vi "设置本机表.vi"(4 "本机表参数":cluster{"有功常数":i32, "无功常数":i32, "输出类型":i32}={"有功常数"=3600000, "无功常数"=3600000, "输出类型"=0}, 5 "串口号":refnum<visa-resource-name>) -> (1 "应答":string)   [LabVIEW 2014]
panel:
  in  "脉冲出口":u8
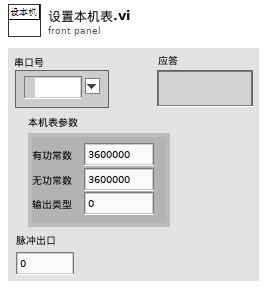
[diagram p1: front panel]
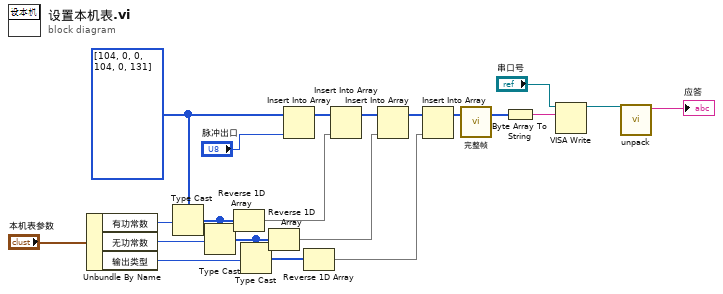
[diagram p0: block diagram]
diagram:
  w9 = u8[] [104, 0, 0, 104, 0, 131]
  n1 = Unbundle By Name("本机表参数") -> ("有功常数"=w12:i32, "无功常数"=w11:i32, "输出类型"=w10:i32)
  n2 = Type Cast(type=w9, x=w12) -> (*(type *) &x=w13:u8[])
  n3 = Type Cast(type=w13, x=w11) -> (*(type *) &x=w14:u8[])
  n4 = Reverse 1D Array(array=w13) -> (reversed array=w8:u8[])
  n5 = Type Cast(type=w14, x=w10) -> (*(type *) &x=w15:u8[])
  n6 = Reverse 1D Array(array=w14) -> (reversed array=w7:u8[])
  n7 = Insert Into Array(array=w9, new element="脉冲出口") -> (w21:u8[])  [unwired: 1 in]
  n8 = Reverse 1D Array(array=w15) -> (reversed array=w6:u8[])
  n9 = Insert Into Array(array=w21, new element=w8) -> (w19:u8[])  [unwired: 1 in]
  n10 = Insert Into Array(array=w19, new element=w7) -> (w18:u8[])  [unwired: 1 in]
  n11 = Insert Into Array(array=w18, new element=w6) -> (w17:u8[])  [unwired: 1 in]
  n12 = call "完整帧.vi"("不完整帧"=w17) -> ("完整帧"=w1:u8[])  [unwired: 2 in]
  n13 = Byte Array To String(unsigned byte array=w1) -> (string=w2:string)
  n14 = VISA Write(VISA resource name="串口号", write buffer=w2) -> (VISA resource name out=w4:refnum<visa-resource-name>)  [unwired: 1 in, 2 out]
  n15 = call "unpack.vi"("串口号输入"=w4) -> ("应答"=→"应答":string)  [unwired: 5 in, 1 out]
